vi "checkdojob.vi"(7 "DO":T1, 10 "sample sn":string[](array[string]), 11 "sample port":refnum<visa-resource-name>[](array[refnum])) -> (0 "DO":string[][](array[string]))   [LabVIEW 2012]
uses:
  globalstatus.vi
  globalreport.vi
panel:
  out "Times":dbl
  in  "Tolerance":dbl
  in  "expect":dbl[](array[numeric])
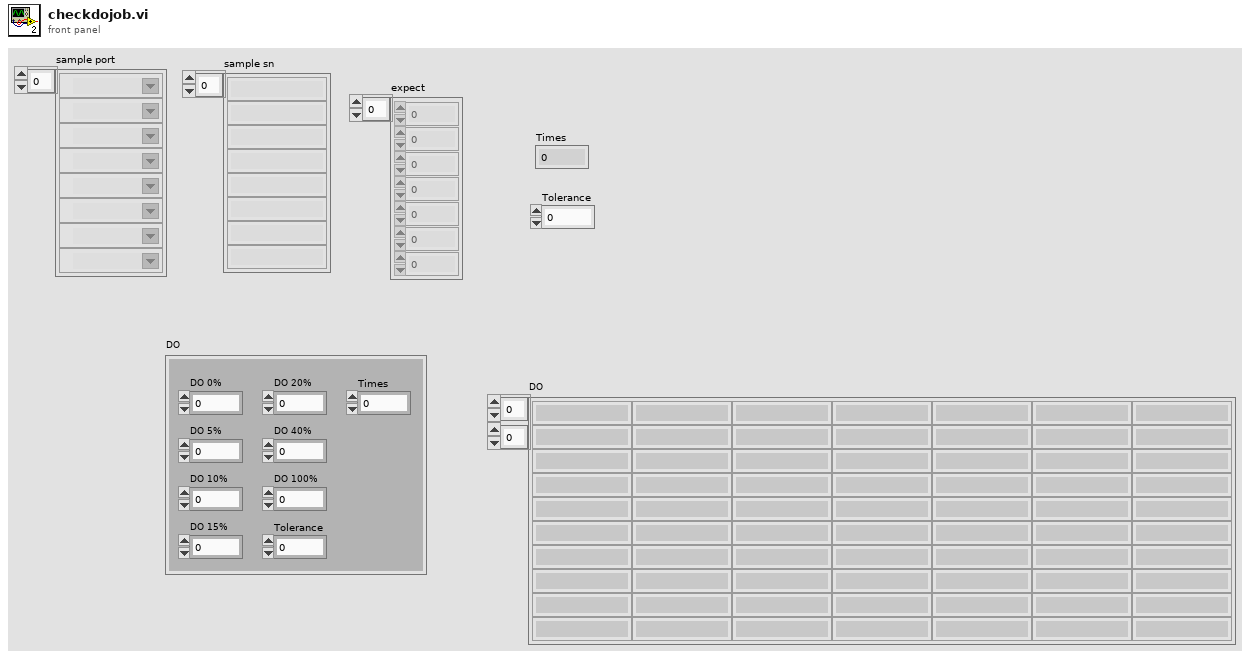
[diagram p1: front panel]
types:
  T1 = cluster{"DO 0%":dbl, "DO 5%":dbl, "DO 10%":dbl, "DO 20%":dbl, "Tolerance":dbl, "DO 15%":dbl, "DO 40%":dbl, "DO 100%":dbl, "Times":dbl}
  T2 = cluster{"PORT":string, "SN":string, "DO 0":string, "DO 1":string, "DO 2":string, "DO 3":string, "DO 4":string, "DO 5":string, "DO 6":string, "result":string, "error":string}[]
  T3 = cluster{"PORT":string, "SN":string, "DO 0":string, "DO 1":string, "DO 2":string, "DO 3":string, "DO 4":string, "DO 5":string, "DO 6":string, string, string}
  T4 = cluster{"PORT":string, "SN":string, "String":string, "String":string, "String":string, "String":string, "String":string, "String":string, "String":string, "result":string, "error":string}
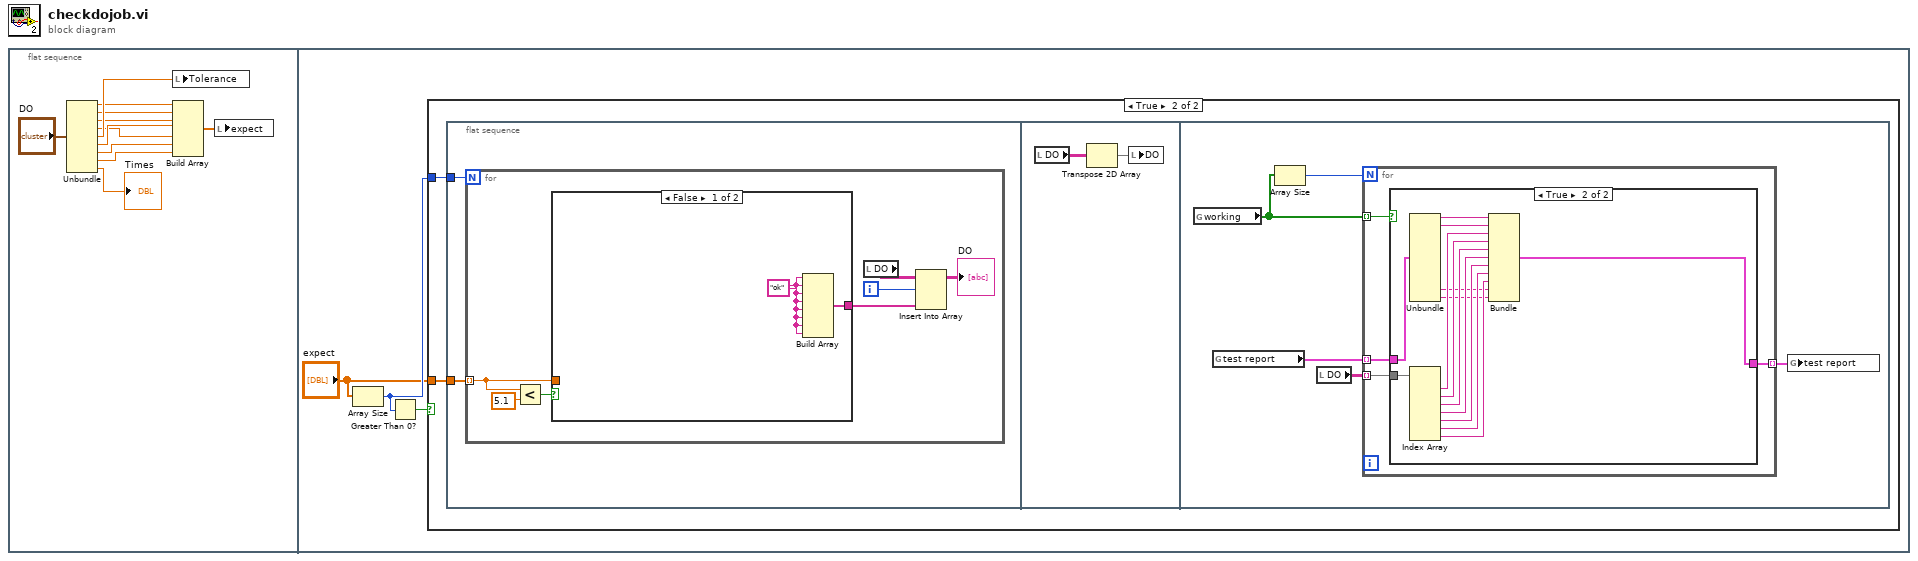
[diagram p0: block diagram]
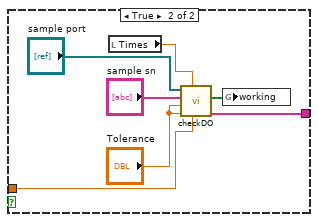
[diagram p3: hidden frame]
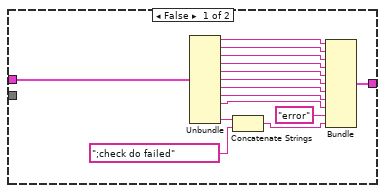
[diagram p4: hidden frame]
diagram:
  n1 = flat-sequence {
    frame #0 {
      n2 = Unbundle("DO") -> ("DO 0%"=w9:dbl, "DO 5%"=w8:dbl, "DO 10%"=w7:dbl, "DO 20%"=w5:dbl, "Tolerance"=w10:dbl, "DO 15%"=w6:dbl, "DO 40%"=w4:dbl, "DO 100%"=w3:dbl, "Times"=→"Times":dbl)
      n3 = local write "Tolerance"(w10) -> ()
      n4 = Build Array(w9, w8, w7, w6, w5, w4, w3) -> (w2:dbl[])
      n5 = local write "expect"(w2) -> ()
    }
    frame #1 {
      n6 = Array Size(array="expect") -> (size(s)=w13:i32)
      n7 = Greater Than 0?(x=w13) -> (x > 0?=w14:bool)
      n8 = case shown="True" w14 {
        tunnel: w13 -> [_ w16]
        tunnel: "expect" -> [_ w15]
        frame False {
        }
        frame True {
          n9 = flat-sequence {
            tunnel: w16 -> [w18]
            tunnel: w15 -> [w17]
            frame #0 {
              n10 = for {
                N: w18 -> [_]
                tunnel: w17 -> [w20] mode=indexing
                i -> [w23]
                n11 = Less?(x=w20, y=5.1) -> (x < y?=w21:bool)
                n12 = case shown="False" w21 {
                  tunnel: w20 -> [_ w32]
                  tunnel: [w26 w28] -> w22
                  frame False {
                    w27 = "ok"
                    n13 = Build Array(w27, w27, w27, w27, w27, w27, w27, w27) -> (w26:string[])
                  }
                  frame True {
                    n14 = local read "Times"() -> (w29:dbl)
                    n15 = call "checkDO.vi"("expect tangent"=w32, "times"=w29, "down"="Tolerance", "up"="Tolerance", "sample sn"="sample sn", "sample port"="sample port") -> ("DO"=w28:string[], "Array"=w30:bool[])  [unwired: 3 in, 1 out]
                    n16 = global write "globalstatus.vi" "working"(w30) -> ()
                  }
                }
                n17 = local read "DO"() -> (w24:string[][])
                n18 = Insert Into Array(array=w24, index (row)=w23, new element=w22) -> (→"DO":string[][])  [unwired: 1 in]
              }
            }
            frame #1 {
              n19 = local read "DO"() -> (w36:string[][])
              n20 = Transpose 2D Array(2D array=w36) -> (transposed array=w35:string[][])
              n21 = local write "DO"(w35) -> ()
            }
            frame #2 {
              n22 = global read "globalstatus.vi" "working"() -> (w37:bool[])
              n23 = global read "globalreport.vi" "test report"() -> (w40:T2)
              n24 = Array Size(array=w37) -> (size(s)=w41:i32)
              n25 = local read "DO"() -> (w38:string[][])
              n26 = for {
                N: w41 -> [_]
                tunnel: w37 -> [w45] mode=indexing
                tunnel: w40 -> [w44] mode=indexing
                tunnel: [w43] -> w39 mode=indexing
                tunnel: w38 -> [w42] mode=indexing
                n27 = case shown="True" w45 {
                  tunnel: w44 -> [w60 w74]
                  tunnel: [w58 w71] -> w43
                  tunnel: w42 -> [_ w70]
                  frame False {
                    n28 = Unbundle(w60) -> ("PORT"=w59:string, "SN"=w57:string, "DO 0"=w56:string, "DO 1"=w55:string, "DO 2"=w54:string, "DO 3"=w53:string, "DO 4"=w52:string, "DO 5"=w51:string, "DO 6"=w50:string, "error"=w46:string)  [unwired: 1 out]
                    n29 = Concatenate Strings(w46, ";check do failed") -> (w47:string)
                    n30 = Bundle("PORT"=w59, "SN"=w57, "DO 0"=w56, "DO 1"=w55, "DO 2"=w54, "DO 3"=w53, "DO 4"=w52, "DO 5"=w51, "DO 6"=w50, "error", w47) -> (w58:T3)  [unwired: 1 in]
                  }
                  frame True {
                    n31 = Unbundle(w74) -> ("PORT"=w73:string, "SN"=w72:string, "result"=w62:string, "error"=w61:string)  [unwired: 7 out]
                    n32 = Index Array(array=w70) -> (element #1=w69:string, element #2=w68:string, element #3=w67:string, element #4=w66:string, element #5=w65:string, element #6=w64:string, element #7=w63:string)  [unwired: 7 in]
                    n33 = Bundle("PORT"=w73, "SN"=w72, "String"=w69, "String"=w68, "String"=w67, "String"=w66, "String"=w65, "String"=w64, "String"=w63, "result"=w62, "error"=w61) -> (w71:T4)  [unwired: 1 in]
                  }
                }
              }
              n34 = global write "globalreport.vi" "test report"(w39) -> ()
            }
          }
        }
      }
    }
  }
